vi "Remove Connection ID.vi"(8 "error in (no error)":errorcluster, 10 "Connection ID":u64, 11 "Web FP In":refnum<class "Web Front Panel.lvclass">) -> (0 "error out":errorcluster)   [LabVIEW 2017, in "Front Panel Publisher.lvlib" / "Web Front Panel.lvclass"]
uses:
  Web Front Panel.lvclass
  Front Panel Manager_class/Protected/Connection ID Methods.ctl
  Front Panel Manager_class/Front Panel Manager.lvclass
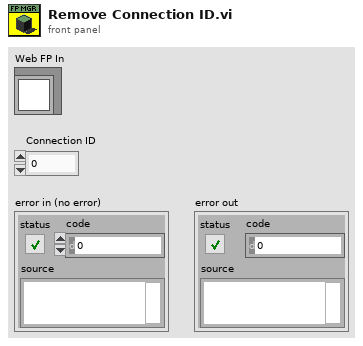
[diagram p1: front panel]
types:
  T1 = typedef "Front Panel Publisher.lvlib/Front Panel Manager.lvclass/Connection ID Methods.ctl" = enum16{"Read Data", "Write Connection ID", "Remove Connection ID"}
  T2 = typedef "Front Panel Publisher.lvlib/Web Front Panel.lvclass/Object Attributes.ctl" = cluster{"VI Identifier":string, "VI Reference":refnum<vi>, "Controls":refnum<class "Object.lvclass">[], "Indicators":refnum<class "Object.lvclass">[], "Decorations":refnum<class "Object.lvclass">[], "VR With Previous Get":refnum<data-value>, "VR With Ring Images":refnum<data-value>}
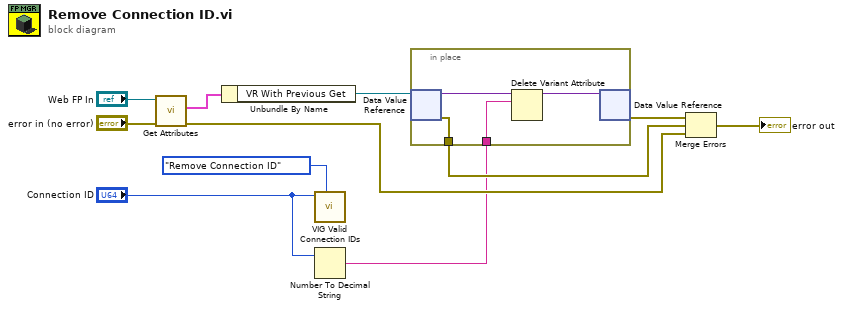
[diagram p0: block diagram]
diagram:
  n1 = call "Get Attributes.vi"("error in (no error)"="error in (no error)", "Web FP In"="Web FP In") -> ("error out"=w4:errorcluster, "Data"=w8:T2)  [unwired: 6 in, 2 out]
  n2 = Unbundle By Name(w8) -> ("VR With Previous Get"=w7:refnum<data-value>)
  n3 = call "VIG Valid Connection IDs.vi"("Method (Read)"=Connection_ID_Methods."Remove Connection ID", "Connection ID"="Connection ID") -> ()  [unwired: 6 in, 4 out]
  n4 = Number To Decimal String(number="Connection ID") -> (decimal integer string=w1:string)  [unwired: 1 in]
  n5 = in-place {
    in-place-border: [w13] -> w3
    in-place-border: w1 -> [w12]
    n6 = in-place-dvr #1(w7) -> (w15:variant, w13:errorcluster)
    n7 = Delete Variant Attribute(6:w12, 7:w15) -> (3:w14:variant)  [unwired: 1 in, 2 out]
    n8 = in-place-dvr #1(w14) -> (w11:errorcluster)  [unwired: 1 out]
  }
  n9 = Merge Errors(w11, w3, w4) -> (→"error out":errorcluster)
